vi "Init TCP.vi"(7 "Error Checking (Full)":T2=enum."Full", 8 "error in (no error)":errorcluster, 11 "VISA resource name":refnum<visa-resource-name>) -> (0 "error out":errorcluster, 2 "Identity":T1, 3 "Session":refnum<class "Session.lvclass">)   [LabVIEW 2024, in "CTI.lvlib" / "VisaComms.lvclass"]
uses:
  VisaComms.lvclass
  Session/Session.lvclass
  Error Reporting.ctl
  Identity.ctl
  C:/Users/nkirchne/Documents/~SANDBOX/Electronics Workflow/build/ForPort/CTI/DeviceComms/DeviceComms.lvclass
  CTI.lvlib
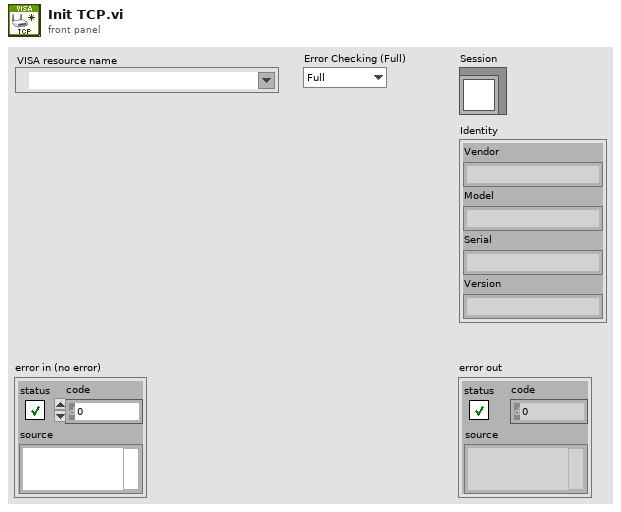
[diagram p1: front panel]
types:
  T1 = typedef "CTI.lvlib/Identity.ctl" = cluster{"Vendor":string, "Model":string, "Serial":string, "Version":string}
  T2 = typedef "CTI.lvlib/Error Reporting.ctl" = enum16{"Minimal", "Moderate", "Full"}
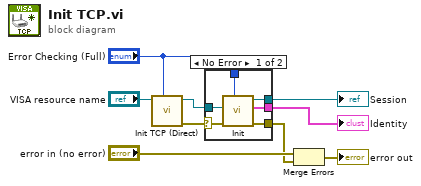
[diagram p0: block diagram]
diagram:
  n1 = call "Init TCP (Direct).vi"("Error Checking (Full)"="Error Checking (Full)", "VISA resource name"="VISA resource name") -> ("error out"=w5:errorcluster, "VisaComms out"=w4:refnum<class "VisaComms.lvclass">)  [unwired: 8 in]
  n2 = case shown="No Error" w5 {
    selector: w5 -> [w12 w16]
    tunnel: [w15 _] -> w6
    tunnel: [w14 w16] -> w7
    tunnel: w4 -> [w13 _]
    tunnel: "Error Checking (Full)" -> [w11 _]
    tunnel: [w10 _] -> w1
    frame No Error {
      n3 = call "Init.vi"("Error Checking (Full)"=w11, "error in (no error)"=w12, "DeviceComms"=w13) -> ("error out"=w14:errorcluster, "Identity"=w10:T1, "Session out"=w15:refnum<class "Session.lvclass">)  [unwired: 6 in]
    }
    frame Error {
    }
  }
  "Session" <- w6
  "Identity" <- w1
  n4 = Merge Errors("error in (no error)", w7) -> (→"error out":errorcluster)
